vi "get_by_index.vi"(9 "frame_stamp":i64, 10 "stream_handle":u64, 11 "path in":path=path "hl2ss_ulm.dll") -> (0 "packet":T1, 1 "packet_handle":u64, 2 "stream_handle":u64, 3 "path out":path)   [LabVIEW 2023]
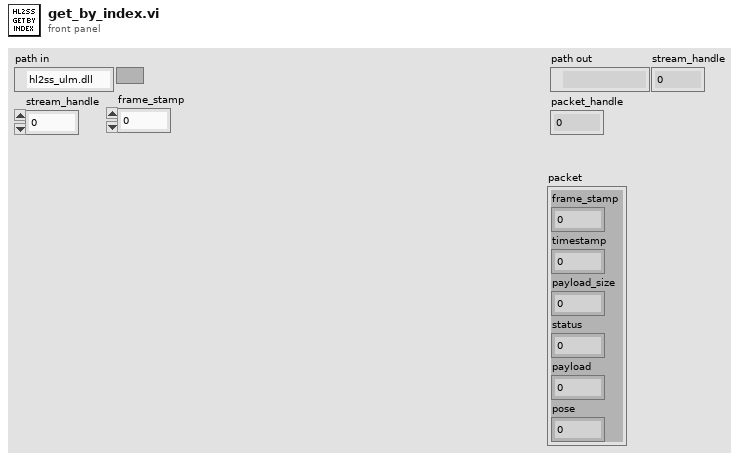
[diagram p1: front panel]
types:
  T1 = cluster{"frame_stamp":i64, "timestamp":u64, "payload_size":u32, "status":i32, "payload":u64, "pose":u64}
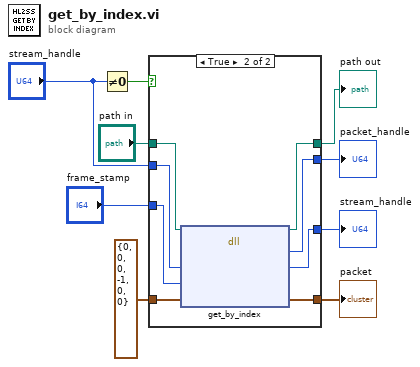
[diagram p0: block diagram]
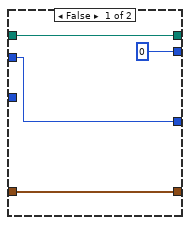
[diagram p2: hidden frame]
diagram:
  n1 = Not Equal To 0?(x="stream_handle") -> (x != 0?=w9:bool)
  n2 = case shown="True" w9 {
    tunnel: "path in" -> [w10 w21]
    tunnel: "stream_handle" -> [w12 w20]
    tunnel: "frame_stamp" -> [_ w19]
    tunnel: T1 {"frame_stamp"=0, "timestamp"=0, "payload_size"=0, "status"=-1, "payload"=0, "pose"=0} ("Cluster") -> [w13 w18]
    tunnel: [w10 w17] -> w5
    tunnel: [u64 0 ("return type") w16] -> w4
    tunnel: [w12 w15] -> w3
    tunnel: [w13 w14] -> w2
    frame False {
    }
    frame True {
      n3 = dll-call lib="C:/Users/jcds/Documents/GitHub/hl2ss/extensions/client_labview/hl2ss_ulm.dll" fn="get_by_index"(path in=w21, "handle"=w20, "frame_stamp"=w19, "packet"=w18) -> (path out=w17:path, "return type"=w16:u64, "handle"=w15:u64, "packet"=w14:T1)  [unwired: 3 in, 1 out]
    }
  }
  "path out" <- w5
  "packet_handle" <- w4
  "stream_handle" <- w3
  "packet" <- w2
